vi "Get-Version-Template.vi"() -> (2 "Commit Reference":string, 3 "Version":string)   [LabVIEW 2019]
doc: "Static VI to get the Version value that was embedded at build-time."
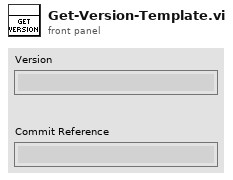
[diagram p1: front panel]
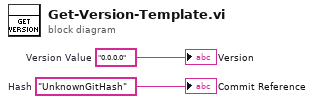
[diagram p0: block diagram]
diagram:
  w1 = "UnknownGitHash"  # Hash
  w2 = "0.0.0.0"  # Version Value
  "Version" <- w2
  "Commit Reference" <- w1
